vi "AlliGator Check Phasor Plot Destination.vi"(9 "Second Plot Name":string, 10 "First Plot Name":string, 11 "Phasor Plot Destination in":T1) -> (1 "Destination Plot Name":string, 3 "Phasor Plot Destination out":T1)   [LabVIEW 2021, in "AlliGator Phasor Graph.lvlib"]
doc: "Checks whether a Phasor Plot Destination is valid (i.e. a valid plot was provided: non empty name) as a destination.\n\nIf not a valid destination, the new plot will be appended to the graph."
uses:
  AlliGator Phasor Graph.lvlib
  AlliGator Phasor Plot Destination.ctl
panel:
  # "see the AlliGator License on the block diagram (Ctrl+E or Window:Show Block Diagram)"
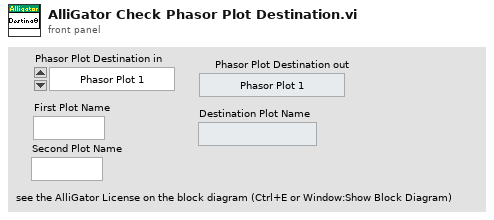
[diagram p1: front panel]
types:
  T1 = typedef "AlliGator Phasor Graph.lvlib/AlliGator Phasor Plot Destination.ctl" = enum32{"Phasor Plot 1", "Phasor Plot 2", "New Phasor Plot"}
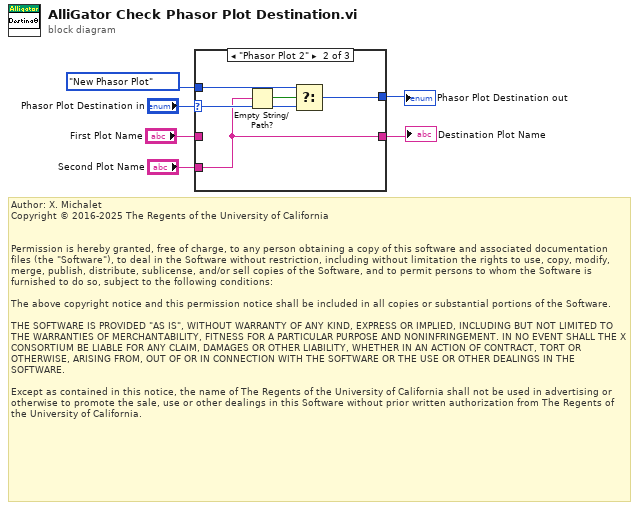
[diagram p0: block diagram]
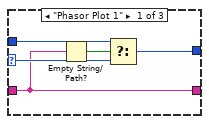
[diagram p2: hidden frame]
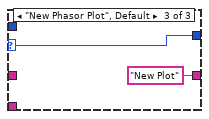
[diagram p3: hidden frame]
diagram:
  # "Author: X. Michalet\nCopyright © 2016-2025 The Regents of the University of California\n \n\nPermission is hereby granted, free of charge, to any person obtaining a copy of this software and associated documentation files (the \"Software\"), to deal in the Software without restriction, including without limitation the rights to use, copy, modify, merge, publish, distribute, sublicense, and/or sell copies of the Software, and to permit persons to whom the Software is furnished to do so, subject to the following conditions:\n\nThe above copyright notice and this permission notice shall be included in all copies or substantial portions of the Software.\n\nTHE SOFTWARE IS PROVIDED \"AS IS\", WITHOUT WARRANTY OF ANY KIND, EXPRESS OR IMPLIED, INCLUDING BUT NOT LIMITED TO THE WARRANTIES OF MERCHANTABILITY, FITNESS FOR A PARTICULAR PURPOSE AND NONINFRINGEMENT. IN NO EVENT SHALL THE X CONSORTIUM BE LIABLE FOR ANY CLAIM, DAMAGES OR OTHER LIABILITY, WHETHER IN AN ACTION OF CONTRACT, TORT OR OTHERWISE, ARISING FROM, OUT OF OR IN CONNECTION WITH THE SOFTWARE OR THE USE OR OTHER DEALINGS IN THE SOFTWARE.\n\nExcept as contained in this notice, the name of The Regents of the University of California shall not be used in advertising or otherwise to promote the sale, use or other dealings in this Software without prior written authorization from The Regents of the University of California."
  n1 = case shown="\"Phasor Plot 2\"" "Phasor Plot Destination in" {
    selector: "Phasor Plot Destination in" -> [w10 w15 w18]
    tunnel: "First Plot Name" -> [w7 _ _]
    tunnel: AlliGator_Phasor_Plot_Destination."New Phasor Plot" ("Phasor Plot Destination in") -> [w9 w14 _]
    tunnel: [w8 w13 w18] -> w4
    tunnel: "Second Plot Name" -> [_ w12 _]
    tunnel: [w7 w12 "New Plot" ("Second Plot Name")] -> w2
    frame "Phasor Plot 1" {
      n2 = Empty String/Path?(string/path=w7) -> (empty?=w11:bool)
      n3 = Select(t=w9, s=w11, f=w10) -> (s? t:f=w8:T1)
    }
    frame "Phasor Plot 2" {
      n4 = Empty String/Path?(string/path=w12) -> (empty?=w16:bool)
      n5 = Select(t=w14, s=w16, f=w15) -> (s? t:f=w13:T1)
    }
    frame "New Phasor Plot", Default {
    }
  }
  "Phasor Plot Destination out" <- w4
  "Destination Plot Name" <- w2
